vi "Get Selective Methods.vi"(8 "error in (no error)":errorcluster, 11 "Methods ListCtrl":refnum<vi>) -> (0 "error out":errorcluster, 3 "Selective Methods":string[](array[string]))   [LabVIEW 2017, in "WebServiceImporter.lvlib" / "Main Panel.lvlib" / "Select Methods.lvlib"]
uses:
  <vilib>/Platform/WebService/Main Panel/Pages/Select Methods/Select Methods.lvlib
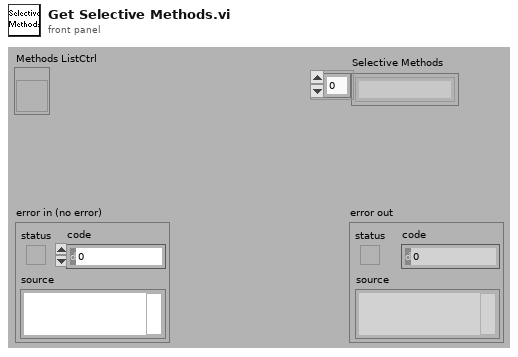
[diagram p1: front panel]
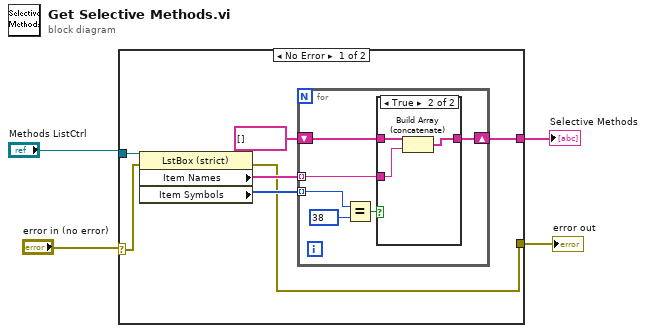
[diagram p0: block diagram]
diagram:
  n1 = case shown="No Error" "error in (no error)" {
    selector: "error in (no error)" -> [w10 w22]
    tunnel: "Methods ListCtrl" -> [w11 _]
    tunnel: [w6 w22] -> w3
    tunnel: [w5 _] -> w2
    frame No Error {
      n2 = property class="LstBox (strict)"(reference=w11, error in=w10) -> (error out=w6:errorcluster, "Item Names"=w9:string[], "Item Symbols"=w8:i32[])  [unwired: 1 out]
      n3 = for {
        tunnel: w9 -> [w14] mode=indexing
        tunnel: w8 -> [w16] mode=indexing
        shift-right: [w12] -> w5
        shift-left: string[] [] -> [w13]
        n4 = Equal?(x=w16, y=38) -> (x = y?=w15:bool)
        n5 = case shown="True" w15 {
          tunnel: w14 -> [_ w21]
          tunnel: w13 -> [w18 w20]
          tunnel: [w18 w19] -> w12
          frame False {
          }
          frame True {
            n6 = Build Array (concatenate)(w20, w21) -> (w19:string[])
          }
        }
      }
    }
    frame Error {
    }
  }
  "Selective Methods" <- w2
  "error out" <- w3
